vi "phy_dpsk_demod.vi"(8 "arity":enum16{"binary", "quadrature"}(ring), 11 "dpsk":cdb[](array[numeric])) -> (3 "bitstream":u8[](array[numeric]))   [LabVIEW 2014]
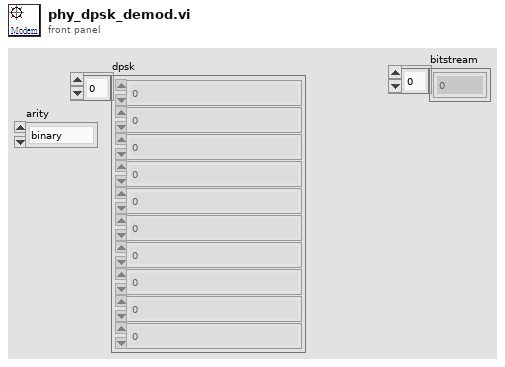
[diagram p1: front panel]
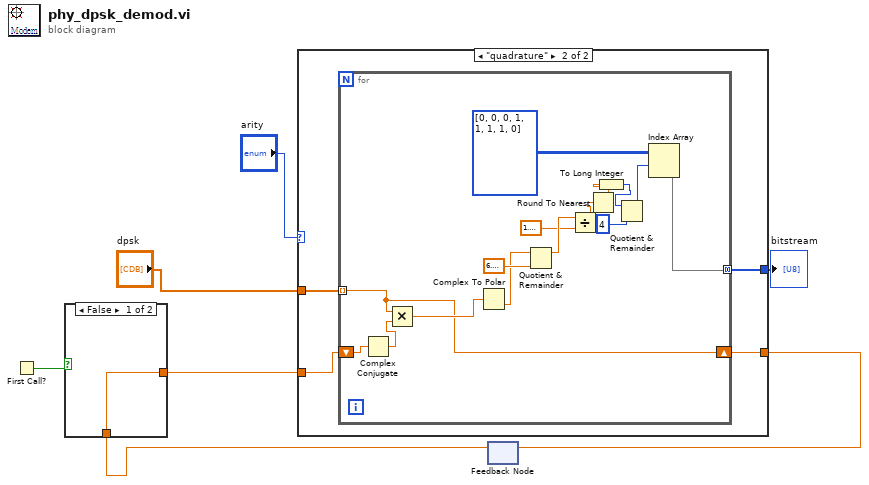
[diagram p0: block diagram]
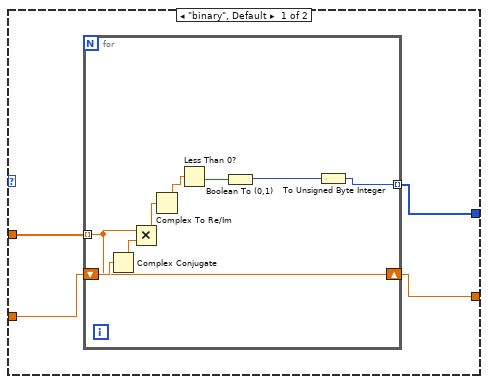
[diagram p2: hidden frame]
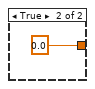
[diagram p3: hidden frame]
diagram:
  n1 = First Call?() -> (First Call?: T/F=w6:bool)
  n2 = feedback #1() -> (w3:cdb)  [unwired: 1 in]
  n3 = case shown="False" w6 {
    tunnel: [w8 0.0 ("Numeric")] -> w5
    tunnel: w3 -> [w8 _]
    frame False {
    }
    frame True {
    }
  }
  n4 = case shown="\"quadrature\"" "arity" {
    tunnel: "dpsk" -> [w12 w25]
    tunnel: w5 -> [w13 w24]
    tunnel: [w10 w23] -> w4
    tunnel: [w11 w22] -> w1
    frame "binary", Default {
      n5 = for {
        shift-right: [w19] -> w10
        shift-left: w13 -> [w21]
        tunnel: w12 -> [w19] mode=indexing
        tunnel: [w14] -> w11 mode=indexing
        n6 = Complex Conjugate(1:w21) -> (0:w20:cdb)
        n7 = Multiply(x=w19, y=w20) -> (x*y=w18:cdb)
        n8 = Complex To Re/Im(x + iy=w18) -> (x=w17:dbl)  [unwired: 1 out]
        n9 = Less Than 0?(x=w17) -> (x < 0?=w16:bool)
        n10 = Boolean To (0,1)(Boolean=w16) -> (0, 1=w15:i16)
        n11 = To Unsigned Byte Integer(number=w15) -> (unsigned 8bit integer=w14:u8)
      }
    }
    frame "quadrature" {
      n12 = for {
        tunnel: w25 -> [w36] mode=indexing
        shift-right: [w36] -> w23
        shift-left: w24 -> [w40]
        tunnel: [w37] -> w22 mode=concatenating
        n13 = Complex Conjugate(1:w40) -> (0:w39:cdb)
        n14 = Multiply(x=w36, y=w39) -> (x*y=w38:cdb)
        n15 = Complex To Polar(r * e^(i*theta)=w38) -> (theta=w26:dbl)  [unwired: 1 out]
        n16 = Quotient & Remainder(x=w26, y=6.283185307179586) -> (x-y*floor(x/y)=w34:dbl)  [unwired: 1 out]
        n17 = Divide(x=w34, y=1.5707963267948966) -> (x/y=w32:dbl)
        n18 = Round To Nearest(number=w32) -> (nearest integer value=w30:dbl)
        n19 = To Long Integer(number=w30) -> (32bit integer=w27:i32)
        n20 = Quotient & Remainder(x=w27, y=4) -> (x-y*floor(x/y)=w28:i32)  [unwired: 1 out]
        n21 = Index Array(array=u8[][] [[0, 0], [0, 1], [1, 1], [1, 0]], index (row)=w28) -> (element=w37:u8[])  [unwired: 1 in]
      }
    }
  }
  "bitstream" <- w1
  n22 = feedback-in #1(w4) -> ()
